vi "Add Users.vi"(8 "error In":errorcluster) -> (0 "error out":errorcluster)   [LabVIEW 2018]
uses:
  Control/Control 7.ctl
panel:
  in  "Stop Button":bool
  in  "Login":bool
  in  "Enum":T1
  in  "Selection":enum16{"VVDN TECH", "Operator", "QA"}(ring)
  in  "Confirm Password":string
  in  "Password":string
  in  "UserName":string
  out "Login":bool
  in  "Password":string
  in  "User Name":string(combo)="VVDN TECH"
  in  "Add User":bool
  in  "Project-Name":string="LensTuning"
  # "ADD USERS"
  # "Admin Login"
  # "User Details"
  # "User Type Selection"
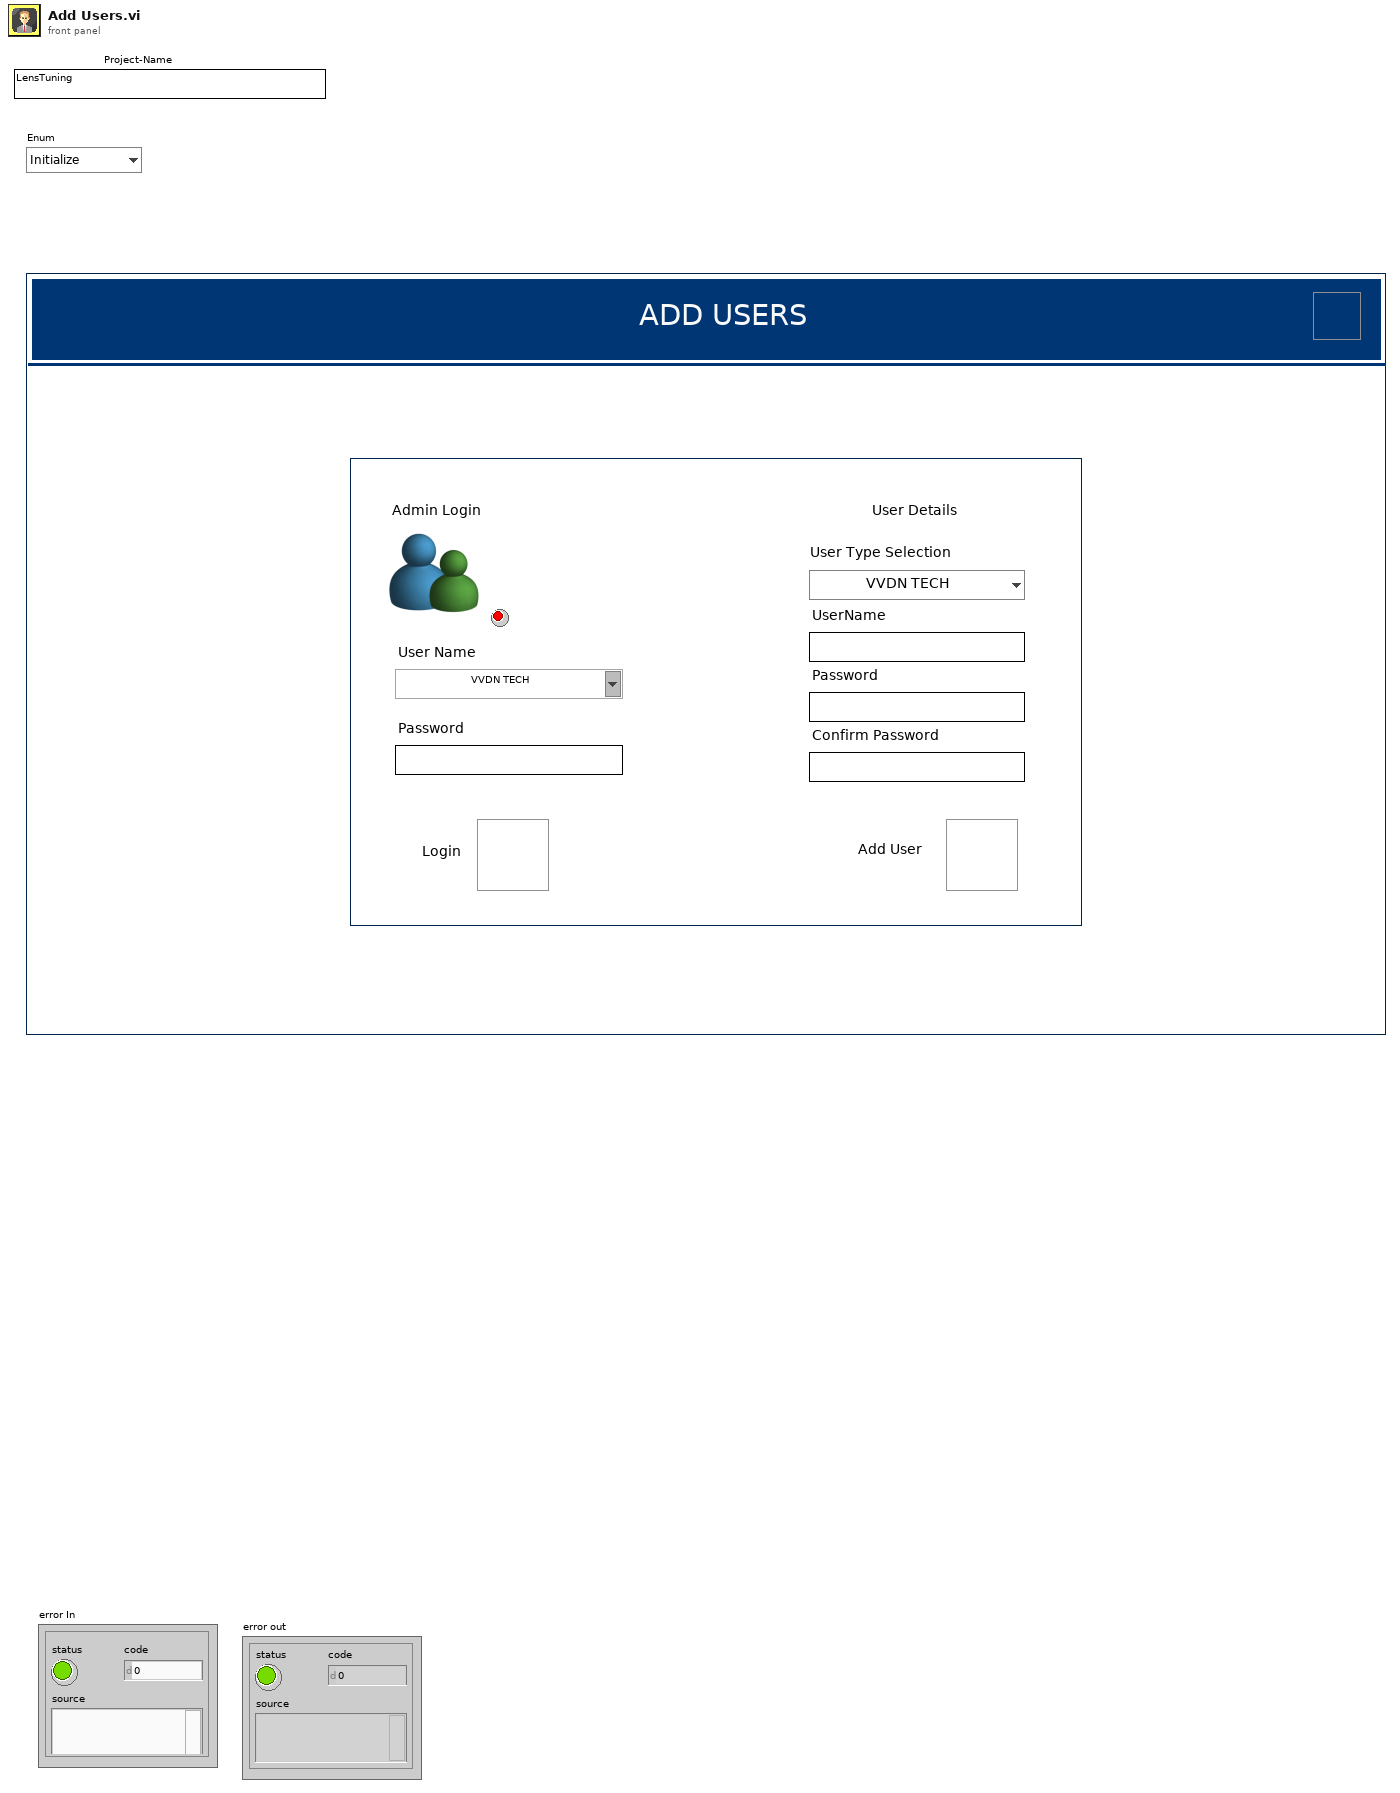
[diagram p1: front panel]
types:
  T1 = typedef "Control 7.ctl" = enum16{"Initialize", "Poll", "Login", "Add User", "Exit"}
  T2 = cluster{"Default User ":string, "Default Password":string, "Default User Type":u16}[]
  T3 = enum32{"Invalid", "Standard", "Closed", "Hidden", "Minimized", "Maximized"}
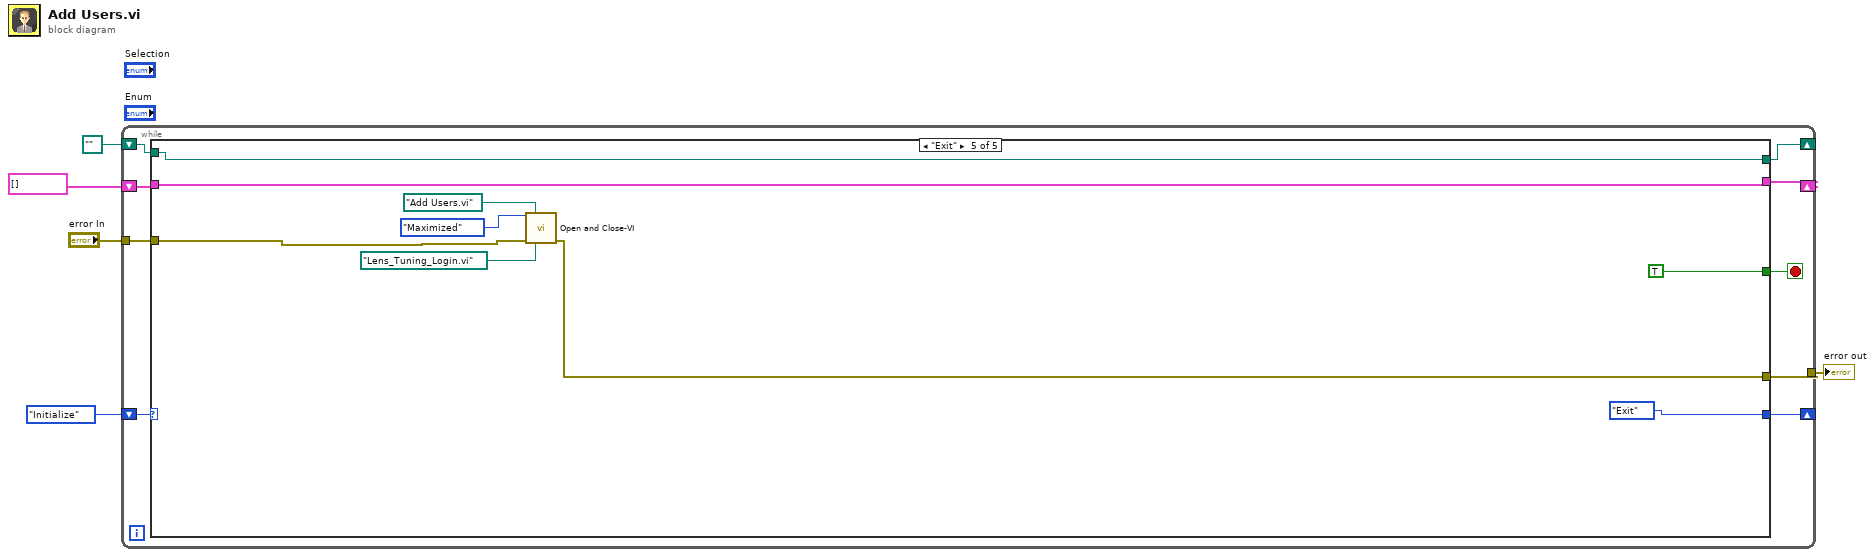
[diagram p0: block diagram]
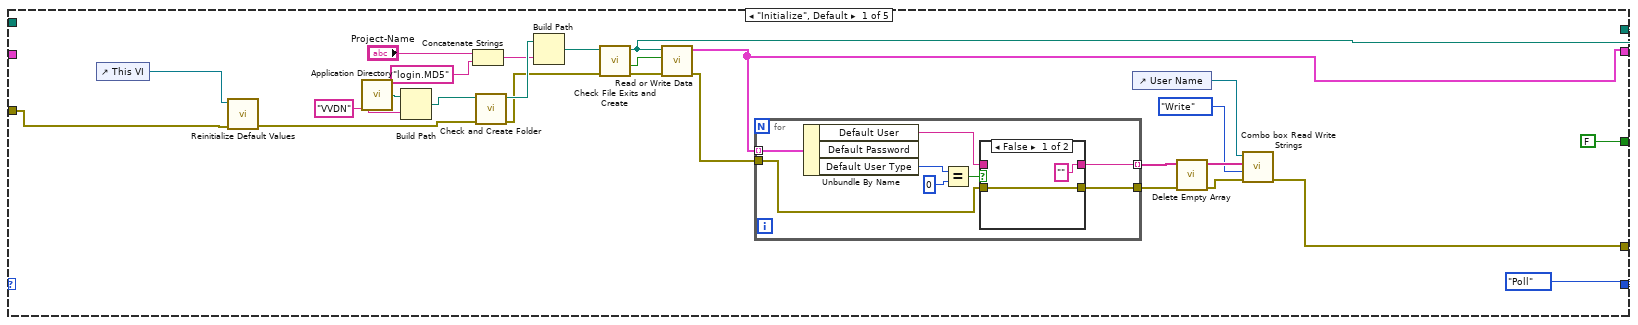
[diagram p2: hidden frame]
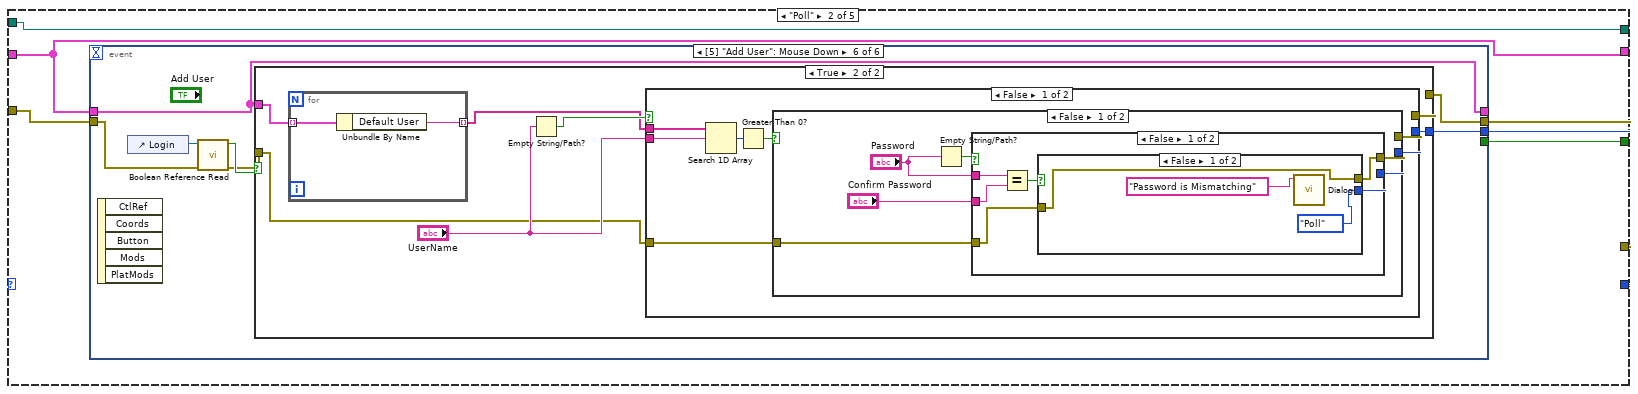
[diagram p4: hidden frame]
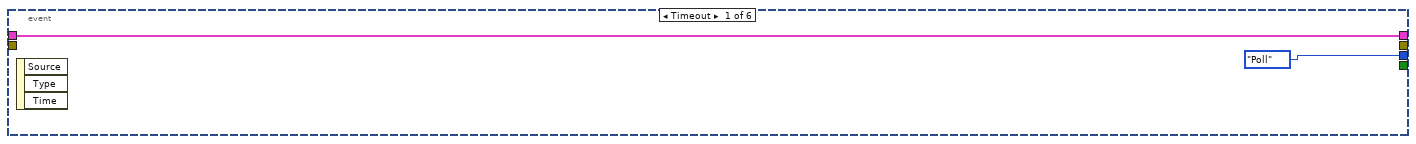
[diagram p5: hidden frame]
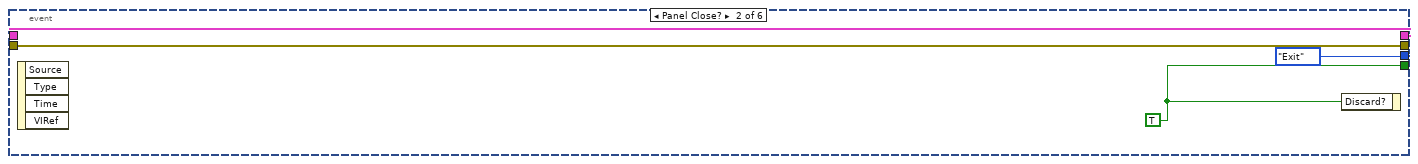
[diagram p6: hidden frame]
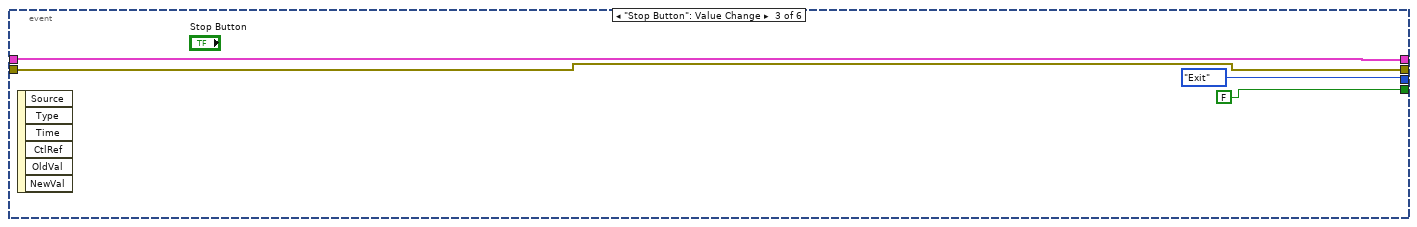
[diagram p7: hidden frame]
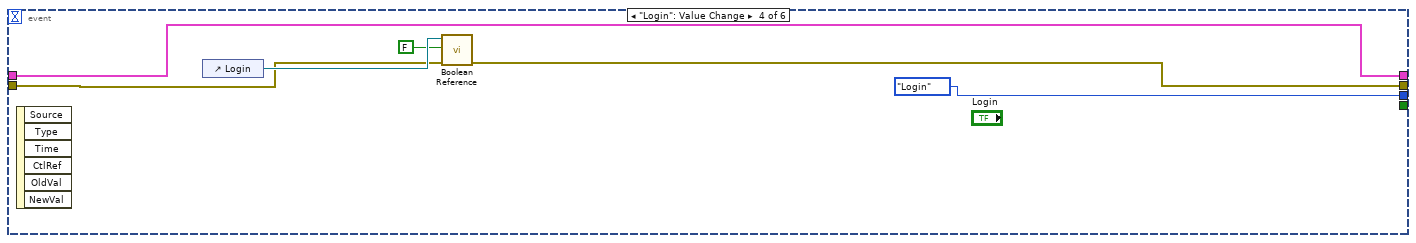
[diagram p8: hidden frame]
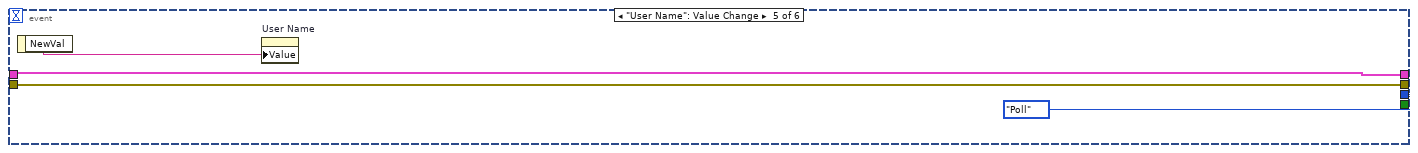
[diagram p9: hidden frame]
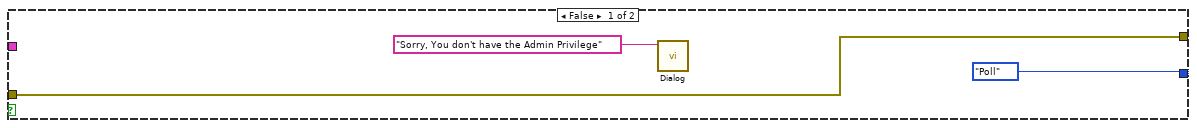
[diagram p10: hidden frame]
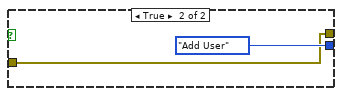
[diagram p11: hidden frame]
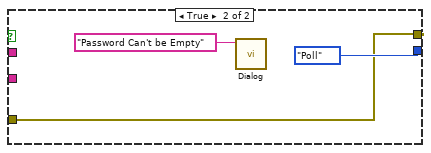
[diagram p12: hidden frame]
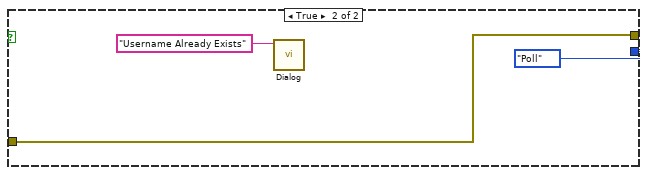
[diagram p13: hidden frame]
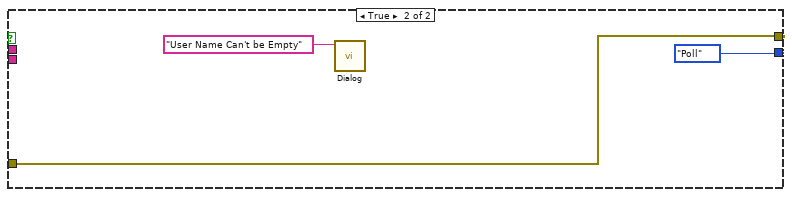
[diagram p14: hidden frame]
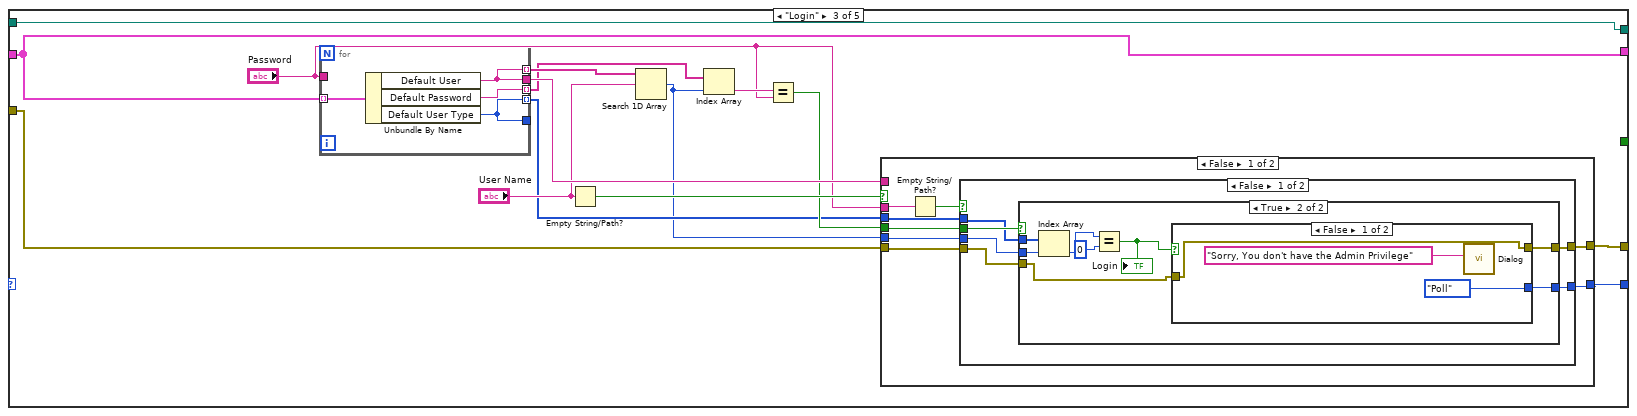
[diagram p15: hidden frame]
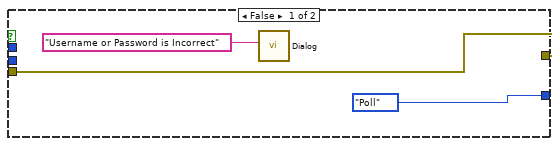
[diagram p16: hidden frame]
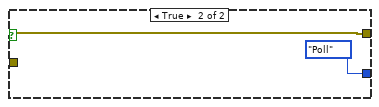
[diagram p17: hidden frame]
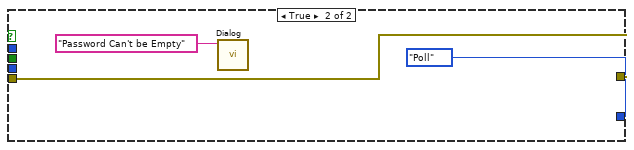
[diagram p18: hidden frame]
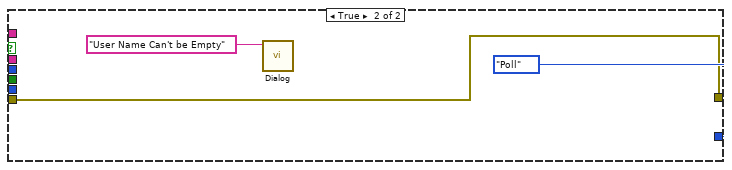
[diagram p19: hidden frame]
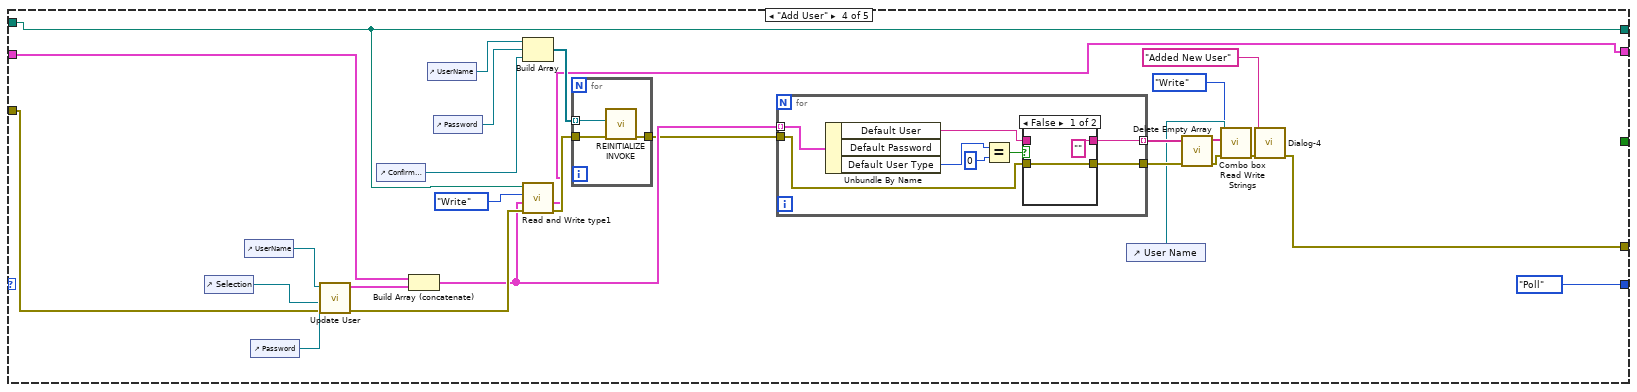
[diagram p20: hidden frame]
diagram:
  n1 = while {
    shift-right: [w10] -> _
    shift-left: Control_7."Initialize" ("Enum") -> [w14]
    tunnel: "error In" -> [w13]
    tunnel: [w12] -> w4
    shift-right: [w6] -> _
    shift-left: T2 [] ("User Details") -> [w11]
    shift-right: [w8] -> _
    shift-left: path "" ("Path Out") -> [w7]
    stop <- w9 stop-if-true
    n2 = case shown="\"Exit\"" w14 {
      tunnel: w13 -> [w17 w58 w145 w207 w235]
      tunnel: [w19 w56 w142 w193 w234] -> w12
      tunnel: w11 -> [_ w57 w139 w205 w228]
      tunnel: [Control_7."Poll" ("Enum") w55 w143 Control_7."Poll" ("Enum") Control_7."Exit" ("Enum")] -> w10
      tunnel: [FALSE ("Discard?") w54 _ _ TRUE ("Discard?")] -> w9
      tunnel: [w27 w53 w140 w208 w229] -> w8
      tunnel: w7 -> [_ w53 w140 w208 w229]
      tunnel: [w26 w57 w139 w194 w228] -> w6
      frame "Initialize", Default {
        n3 = control-ref of="This VI"() -> (w15:refnum<vi>)
        n4 = call "Reinitialize Default Values.vi"("error in (no error)"=w17, "VI in"=w15) -> ("error out"=w16:errorcluster)  [unwired: 9 in]
        n5 = call <vilib>:"Application Directory.vi"() -> ("Application Directory"=w38:path)
        n6 = Build Path(base path=w38, name or relative path="VVDN") -> (appended path=w34:path)
        n7 = Concatenate Strings("Project-Name", "login.MD5" ("string")) -> (w32:string)
        n8 = call "Check and Create Folder.vi"("error in (no error)"=w16, "Path In"=w34) -> ("error out"=w31:errorcluster, "Path Out"=w33:path)  [unwired: 7 in, 1 out]
        n9 = Build Path(base path=w33, name or relative path=w32) -> (appended path=w30:path)
        n10 = call "Check File Exits and Create.vi"("error in"=w31, "Path In"=w30) -> ("error out"=w39:errorcluster, "file exists?"=w40:bool, "Path Out"=w27:path)  [unwired: 6 in, 1 out]
        n11 = call "Read or Write Data.vi"("error in"=w39, "file exists?"=w40, "Path Out"=w27) -> ("error out"=w25:errorcluster, "User Details"=w26:T2)  [unwired: 7 in]
        n12 = for {
          tunnel: w26 -> [w48] mode=indexing
          tunnel: w25 -> [w43]
          tunnel: [w42] -> w24 mode=indexing
          tunnel: [w41] -> w23
          n13 = Unbundle By Name(w48) -> ("Default User"=w44:string, "Default User Type"=w47:u16)  [unwired: 1 out]
          n14 = Equal?(x=w47, y=u16 0) -> (x = y?=w45:bool)
          n15 = case shown="False" w45 {
            tunnel: w44 -> [_ w52]
            tunnel: ["" ("Default User") w52] -> w42
            tunnel: [w49 w51] -> w41
            tunnel: w43 -> [w49 w51]
            frame False {
            }
            frame True {
            }
          }
        }
        n16 = control-ref of="User Name"() -> (w22:refnum<vi>)
        n17 = call "Delete Empty Array.vi"("error in"=w23, "Array in"=w24) -> ("error out"=w20:errorcluster, "Array out"=w21:string[])  [unwired: 8 in]
        n18 = call "Combo box Read Write Strings.vi"("error in (no error)"=w20, "Enum"=enum16{"Read", "Write"}."Write", "Strings []"=w21, "ComboBox in"=w22) -> ("error out"=w19:errorcluster)  [unwired: 6 in, 1 out]
      }
      frame "Poll" {
        n19 = event shown="[5] \"Add User\": Mouse Down" {
          selector: _ -> [_ _ _ _ _ _]
          dyn-events: _ -> [_ _ _ _ _ _]
          timeout: _ -> [_ _ _ _ _ _]
          tunnel: w58 -> [_ w64 w66 w70 w77 w82]
          tunnel: w57 -> [w59 w63 w68 w74 w75 w84]
          tunnel: [w59 w63 w68 w74 w75 w84] -> _
          tunnel: [_ w64 w66 w69 w77 w83] -> w56
          tunnel: [Control_7."Poll" ("Enum") Control_7."Exit" ("Enum") Control_7."Exit" ("Enum") Control_7."Login" ("Enum") Control_7."Poll" ("Enum") w85] -> w55
          tunnel: [_ w62 FALSE ("Discard?") _ _ _] -> w54
          event Timeout {
            n20 = event-data() -> ()  [unwired: 1 in, 3 out]
          }
          event Panel Close? {
            w62 = TRUE ("Discard?")
            n21 = event-data() -> ()  [unwired: 1 in, 4 out]
            n22 = event-data("Discard?"=w62) -> ()  [unwired: 1 in, 1 out]
          }
          event "Stop Button": Value Change {
            n23 = event-data() -> ()  [unwired: 1 in, 6 out]
          }
          event "Login": Value Change {
            n24 = event-data() -> ()  [unwired: 1 in, 6 out]
            n25 = control-ref of="Login"() -> (w72:refnum<vi>)
            n26 = call "Boolean Reference.vi"("error in"=w70, "Value"=FALSE, "Boolean in"=w72) -> ("error out"=w69:errorcluster)  [unwired: 8 in]
          }
          event "User Name": Value Change {
            n27 = event-data() -> ("NewVal"=w78:string)  [unwired: 1 in]
            n28 = property on="User Name" class="CmbBox"("Value"=w78) -> ()  [unwired: 2 in, 2 out]
          }
          event "Add User": Mouse Down {
            n29 = event-data() -> ()  [unwired: 1 in, 5 out]
            n30 = control-ref of="Login"() -> (w81:refnum<vi>)
            n31 = call "Boolean Reference Read.vi"("error in (no error)"=w82, "Boolean in"=w81) -> ("error out"=w79:errorcluster, "Value"=w80:bool)  [unwired: 8 in]
            n32 = case shown="True" w80 {
              tunnel: [Control_7."Poll" ("Enum") w94] -> w85
              tunnel: w84 -> [_ w93]
              tunnel: w79 -> [w87 w90]
              tunnel: [w87 w89] -> w83
              frame False {
                n33 = call "Dialog.vi"("Status"="Sorry, You don't have the Admin Privilege") -> ()  [unwired: 10 in, 1 out]
              }
              frame True {
                n34 = for {
                  tunnel: w93 -> [w97] mode=indexing
                  tunnel: [w96] -> w92 mode=indexing
                  n35 = Unbundle By Name(w97) -> ("Default User"=w96:string)
                }
                n36 = Empty String/Path?(string/path="UserName") -> (empty?=w95:bool)
                n37 = case shown="False" w95 {
                  tunnel: [w102 Control_7."Poll" ("Enum")] -> w94
                  tunnel: w92 -> [w99 _]
                  tunnel: "UserName" -> [w98 _]
                  tunnel: w90 -> [w101 w128]
                  tunnel: [w100 w128] -> w89
                  frame False {
                    n38 = Search 1D Array(1D array=w99, element=w98) -> (index of element=w104:i32)  [unwired: 1 in]
                    n39 = Greater Than 0?(x=w104) -> (x > 0?=w103:bool)
                    n40 = case shown="False" w103 {
                      tunnel: [w109 Control_7."Poll" ("Enum")] -> w102
                      tunnel: w101 -> [w106 w125]
                      tunnel: [w105 w125] -> w100
                      frame False {
                        n41 = Empty String/Path?(string/path="Password") -> (empty?=w110:bool)
                        n42 = case shown="False" w110 {
                          tunnel: [w113 Control_7."Poll" ("Enum")] -> w109
                          tunnel: "Password" -> [w116 _]
                          tunnel: "Confirm Password" -> [w115 _]
                          tunnel: w106 -> [w112 w122]
                          tunnel: [w111 w122] -> w105
                          frame False {
                            n43 = Equal?(x=w116, y=w115) -> (x = y?=w114:bool)
                            n44 = case shown="False" w114 {
                              tunnel: [Control_7."Poll" ("Enum") Control_7."Add User" ("Enum")] -> w113
                              tunnel: w112 -> [w117 w120]
                              tunnel: [w117 w120] -> w111
                              frame False {
                                n45 = call "Dialog.vi"("Status"="Password is Mismatching") -> ()  [unwired: 10 in, 1 out]
                              }
                              frame True {
                              }
                            }
                          }
                          frame True {
                            n46 = call "Dialog.vi"("Status"="Password Can't be Empty") -> ()  [unwired: 10 in, 1 out]
                          }
                        }
                      }
                      frame True {
                        n47 = call "Dialog.vi"("Status"="Username Already Exists") -> ()  [unwired: 10 in, 1 out]
                      }
                    }
                  }
                  frame True {
                    n48 = call "Dialog.vi"("Status"="User Name Can't be Empty") -> ()  [unwired: 10 in, 1 out]
                  }
                }
              }
            }
          }
        }
      }
      frame "Login" {
        n49 = for {
          tunnel: w139 -> [w149] mode=indexing
          tunnel: [w148] -> w141
          tunnel: "Password" -> [_]
          tunnel: [w146] -> _
          tunnel: [w148] -> w138 mode=indexing
          tunnel: [w147] -> w137 mode=indexing
          tunnel: [w146] -> w132 mode=indexing
          n50 = Unbundle By Name(w149) -> ("Default User"=w148:string, "Default Password"=w147:string, "Default User Type"=w146:u16)
        }
        n51 = Empty String/Path?(string/path="User Name") -> (empty?=w144:bool)
        n52 = Search 1D Array(1D array=w138, element="User Name") -> (index of element=w131:i32)  [unwired: 1 in]
        n53 = Index Array(array=w137, index=w131) -> (element=w136:string)
        n54 = Equal?(x=w136, y="Password") -> (x = y?=w134:bool)
        n55 = case shown="False" w144 {
          tunnel: w145 -> [w155 w183]
          tunnel: [w153 Control_7."Poll" ("Enum")] -> w143
          tunnel: [w154 w183] -> w142
          tunnel: w141 -> [_ _]
          tunnel: "Password" -> [w157 _]
          tunnel: w131 -> [w152 _]
          tunnel: w134 -> [w151 _]
          tunnel: w132 -> [w150 _]
          frame False {
            n56 = Empty String/Path?(string/path=w157) -> (empty?=w156:bool)
            n57 = case shown="False" w156 {
              tunnel: w155 -> [w163 w182]
              tunnel: [w162 w182] -> w154
              tunnel: [w161 Control_7."Poll" ("Enum")] -> w153
              tunnel: w152 -> [w160 _]
              tunnel: w151 -> [w159 _]
              tunnel: w150 -> [w158 _]
              frame False {
                n58 = case shown="True" w159 {
                  tunnel: w163 -> [w165 w173]
                  tunnel: [w165 w172] -> w162
                  tunnel: [Control_7."Poll" ("Enum") w171] -> w161
                  tunnel: w160 -> [_ w169]
                  tunnel: w158 -> [_ w168]
                  frame False {
                    n59 = call "Dialog.vi"("Status"="Username or Password is Incorrect") -> ()  [unwired: 10 in, 1 out]
                  }
                  frame True {
                    n60 = Index Array(array=w168, index=w169) -> (element=w167:u16)
                    n61 = Equal?(x=w167, y=u16 0) -> (x = y?=w170:bool)
                    "Login" <- w170
                    n62 = case shown="False" w170 {
                      tunnel: w173 -> [w176 w179]
                      tunnel: [w176 w179] -> w172
                      tunnel: [Control_7."Poll" ("Enum") Control_7."Poll" ("Enum")] -> w171
                      frame False {
                        n63 = call "Dialog.vi"("Status"="Sorry, You don't have the Admin Privilege") -> ()  [unwired: 10 in, 1 out]
                      }
                      frame True {
                      }
                    }
                  }
                }
              }
              frame True {
                n64 = call "Dialog.vi"("Status"="Password Can't be Empty") -> ()  [unwired: 10 in, 1 out]
              }
            }
          }
          frame True {
            n65 = call "Dialog.vi"("Status"="User Name Can't be Empty") -> ()  [unwired: 10 in, 1 out]
          }
        }
      }
      frame "Add User" {
        n66 = control-ref of="Selection"() -> (w186:refnum<vi>)
        n67 = control-ref of="UserName"() -> (w211:refnum<vi>)
        n68 = control-ref of="Password"() -> (w210:refnum<vi>)
        n69 = call "Update User.vi"("error In"=w207, "Selection"=w186, "Password"=w210, "String in"=w211) -> ("error Out"=w206:errorcluster, "User Details"=w204:T2)  [unwired: 6 in]
        n70 = control-ref of="Confirm Password"() -> (w201:refnum<vi>)
        n71 = Build Array (concatenate)(w205, w204) -> (w196:T2)
        n72 = control-ref of="UserName"() -> (w203:refnum<vi>)
        n73 = control-ref of="Password"() -> (w202:refnum<vi>)
        n74 = Build Array(w203, w202, w201) -> (w200:refnum<vi>[])
        n75 = call "Read and Write type1.vi"("error in"=w206, "IN"=w196, "Enum"=enum16{"Init", "Read", "Write"}."Write", "Path Out"=w208) -> ("error out"=w199:errorcluster, "OUT"=w194:T2)  [unwired: 6 in]
        n76 = for {
          tunnel: w200 -> [w227] mode=indexing
          tunnel: w199 -> [w226]
          tunnel: [w225] -> w195
          n77 = call "REINITIALIZE INVOKE.vi"("error in (no error)"=w226, "Str Refnum"=w227) -> ("error out"=w225:errorcluster)  [unwired: 9 in]
        }
        n78 = for {
          tunnel: w196 -> [w220] mode=indexing
          tunnel: w195 -> [w215]
          tunnel: [w214] -> w198 mode=indexing
          tunnel: [w213] -> w197
          n79 = Unbundle By Name(w220) -> ("Default User"=w216:string, "Default User Type"=w219:u16)  [unwired: 1 out]
          n80 = Equal?(x=w219, y=u16 0) -> (x = y?=w217:bool)
          n81 = case shown="False" w217 {
            tunnel: w216 -> [_ w224]
            tunnel: ["" ("Default User") w224] -> w214
            tunnel: [w221 w223] -> w213
            tunnel: w215 -> [w221 w223]
            frame False {
            }
            frame True {
            }
          }
        }
        n82 = control-ref of="User Name"() -> (w191:refnum<vi>)
        n83 = call "Delete Empty Array.vi"("error in"=w197, "Array in"=w198) -> ("error out"=w189:errorcluster, "Array out"=w187:string[])  [unwired: 8 in]
        n84 = call "Combo box Read Write Strings.vi"("error in (no error)"=w189, "Enum"=enum16{"Read", "Write"}."Write", "Strings []"=w187, "ComboBox in"=w191) -> ("error out"=w188:errorcluster)  [unwired: 6 in, 1 out]
        n85 = call "Dialog-4.vi"("error in"=w188, "Status"="Added New User") -> ("error out"=w193:errorcluster)  [unwired: 8 in, 1 out]
      }
      frame "Exit" {
        n86 = call "Open and Close-VI.vi"("State"=T3."Maximized", "Close VI"=path "Add Users.vi", "error in"=w235, "Open VI"=path "Lens_Tuning_Login.vi") -> ("error out"=w234:errorcluster)  [unwired: 11 in]
      }
    }
  }
  "error out" <- w4
